vi "runViComplex.vi"(8 "error in (no error)":errorcluster) -> (0 "error out":errorcluster, 3 "variantOut":variant)   [LabVIEW 2018]
doc: "Run the vi wil the complex inputs and outputs."
panel:
  in  "imag":dbl
  in  "real":dbl
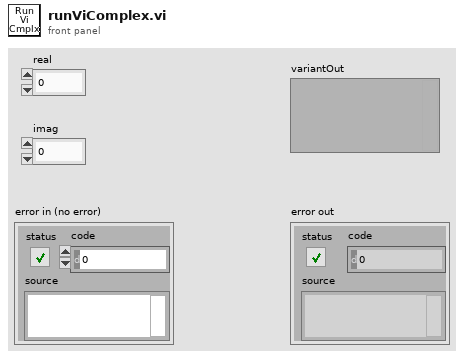
[diagram p1: front panel]
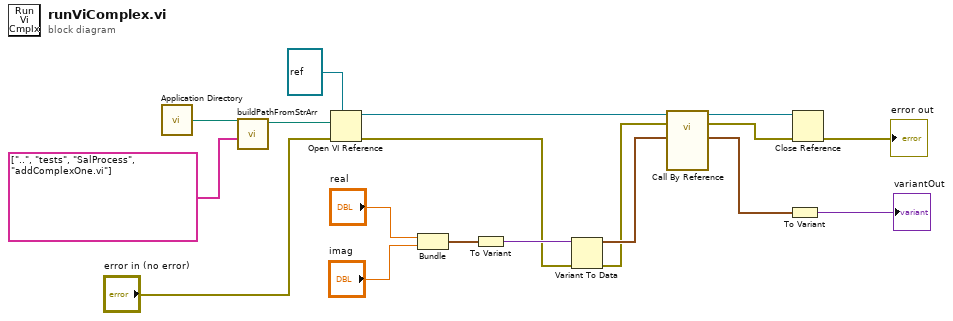
[diagram p0: block diagram]
diagram:
  n1 = call <vilib>:"Application Directory.vi"() -> ("Application Directory"=w18:path)
  n2 = call "buildPathFromStrArr.vi"("String Array"=string[] ["..", "tests", "SalProcess", "addComplexOne.vi"], "Root Path"=w18) -> ("Absolute Path"=w16:path)  [unwired: 9 in]
  n3 = Open VI Reference(type specifier VI Refnum (for type only)=refnum<vi> refnum, vi path=w16, error in (no error)="error in (no error)") -> (vi reference=w13:refnum<vi>, error out=w2:errorcluster)  [unwired: 3 in]
  n4 = Bundle("real"="real", "imag"="imag") -> (w5:cluster{"real":dbl, "imag":dbl})  [unwired: 1 in]
  n5 = To Variant(anything=w5) -> (Variant=w3:variant)
  n6 = Variant To Data(error in=w2, Variant=w3) -> (data=w4:cluster{"real":dbl, "imag":dbl}, error out=w1:errorcluster)  [unwired: 1 in]
  n7 = call-by-ref "?"(reference=w13, error in=w1, "input"=w4) -> (reference out=w12:refnum<vi>, error out=w11:errorcluster, "output"=w8:cluster{"real":dbl, "imag":dbl})  [unwired: 9 in, 1 out]
  n8 = To Variant(anything=w8) -> (Variant=→"variantOut":variant)
  n9 = Close Reference(reference=w12, error in (no error)=w11) -> (error out=→"error out":errorcluster)
